vi "drawball.vi"(6 "new picture in":picture, 9 "reference 2":refnum<vi>, 10 "reference":refnum<vi>, 11 "Digital in":refnum<vi>) -> (3 "new picture":picture)   [LabVIEW 2016]
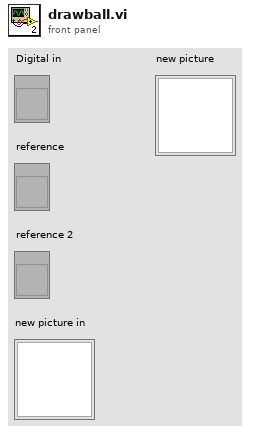
[diagram p1: front panel]
types:
  T1 = cluster{"Width":u16, "Style":enum32{"Solid", "Dash", "Dot", "DashDot", "DashDotDot"}}
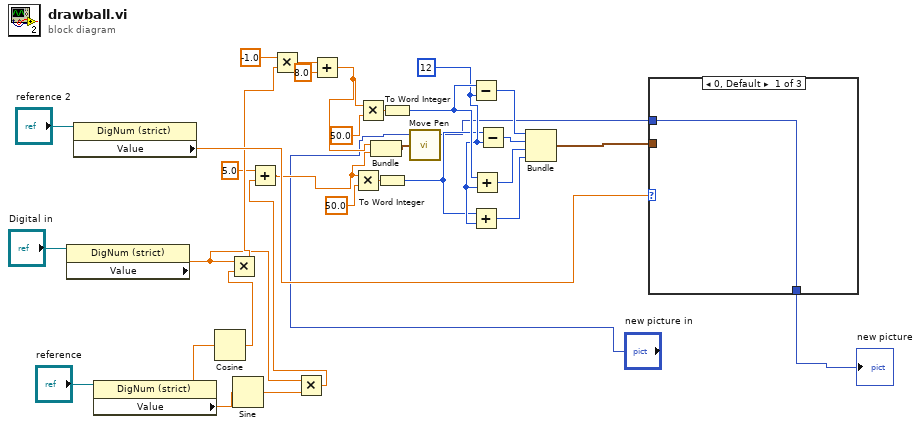
[diagram p0: block diagram]
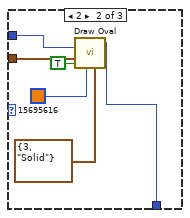
[diagram p2: hidden frame]
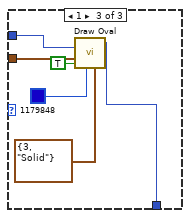
[diagram p3: hidden frame]
diagram:
  w11 = i16 12 ("Waypoint \nSize")
  n1 = property class="DigNum (strict)"(reference="Digital in") -> ("Value"=w28:dbl)  [unwired: 1 in, 2 out]
  n2 = property class="DigNum (strict)"(reference="reference 2") -> ("Value"=w31:dbl)  [unwired: 1 in, 2 out]
  n3 = property class="DigNum (strict)"(reference="reference") -> ("Value"=w25:dbl)  [unwired: 1 in, 2 out]
  n4 = Cosine(x=w25) -> (cos(x)=w27:dbl)
  n5 = Multiply(x=w28, y=w27) -> (x*y=w30:dbl)
  n6 = Sine(x=w25) -> (sin(x)=w26:dbl)
  n7 = Multiply(x=-1.0, y=w30) -> (x*y=w19:dbl)
  n8 = Multiply(x=w28, y=w26) -> (x*y=w29:dbl)
  n9 = Add(x=5.0, y=w29) -> (x+y=w23:dbl)
  n10 = Add(x=w19, y=8.0) -> (x+y=w22:dbl)
  n11 = Multiply(x=w23, y=50.0) -> (x*y=w10:dbl)
  n12 = Multiply(x=w22, y=50.0) -> (x*y=w13:dbl)
  n13 = Bundle(w22, w23) -> (w6:cluster{dbl, dbl})  [unwired: 1 in]
  n14 = To Word Integer(number=w10) -> (16bit integer=w8:i16)
  n15 = To Word Integer(number=w13) -> (16bit integer=w12:i16)
  n16 = call <vilib>:"Move Pen.vi"("new position"=w6, "picture"="new picture in") -> ("new picture"=w5:picture)  [unwired: 3 in]
  n17 = Subtract(x=w12, y=w11) -> (x-y=w18:i16)
  n18 = Add(x=w8, y=w11) -> (x+y=w15:i16)
  n19 = Add(x=w12, y=w11) -> (x+y=w16:i16)
  n20 = Subtract(x=w8, y=w11) -> (x-y=w17:i16)
  n21 = Bundle(w18, w17, w16, w15) -> (w7:cluster{i16, i16, i16, i16})  [unwired: 1 in]
  n22 = case shown="0, Default" w31 {
    tunnel: [w33 w39 w45] -> w32
    tunnel: w5 -> [w33 w37 w43]
    tunnel: w7 -> [_ w36 w42]
    frame 0, Default {
    }
    frame 2 {
      n23 = call <vilib>:"Draw Oval.vi"("picture"=w37, "rect"=w36, "fill?(F)"=TRUE, "color(black)"=u32 15695616, "pen"=T1 {"Width"=3, "Style"=enum."Solid"}) -> ("new picture"=w39:picture)  [unwired: 4 in]
    }
    frame 1 {
      n24 = call <vilib>:"Draw Oval.vi"("picture"=w43, "rect"=w42, "fill?(F)"=TRUE, "color(black)"=u32 1179848, "pen"=T1 {"Width"=3, "Style"=enum."Solid"}) -> ("new picture"=w45:picture)  [unwired: 4 in]
    }
  }
  "new picture" <- w32
